vi "MoAgSy_AgentBase_MSGhandler_wrap.vi"(0 "HGF_Agent in":refnum<class "MoAgSy_AgentBase.lvclass">, 2 "MoAgSy_Message":refnum<class "MoAgSy_Message.lvclass">, 5 "error in (no error)":errorcluster) -> (14 "HGF_Agent out":refnum<class "MoAgSy_AgentBase.lvclass">, 19 "error out":errorcluster)   [LabVIEW 2009, in "MoAgSy_Base.lvlib" / "MoAgSy_AgentBase.lvclass"]
uses:
  MoAgSy_AgentBase.lvclass
  MoAgSy_Message/MoAgSy_Message.lvclass
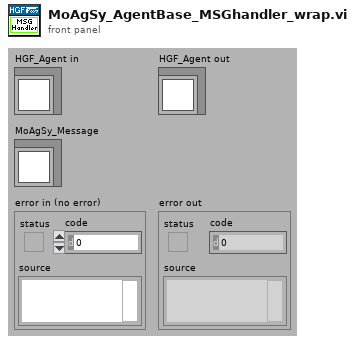
[diagram p1: front panel]
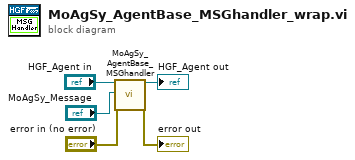
[diagram p0: block diagram]
diagram:
  n1 = call-dynamic "MoAgSy_AgentBase_MSGhandler.vi"("HGF_Agent in"="HGF_Agent in", "MoAgSy_Message"="MoAgSy_Message", "error in (no error)"="error in (no error)") -> ("HGF_Agent out"=→"HGF_Agent out":refnum<class "MoAgSy_AgentBase.lvclass">, "error out"=→"error out":errorcluster)  [unwired: 15 in]
